vi "counter.vi"(7 "Fun":enum16{"Count", "Init"}(ring), 10 "INIT VALUE":dbl format="%#_13g") -> (2 "Numeric":dbl)   [LabVIEW 2015]
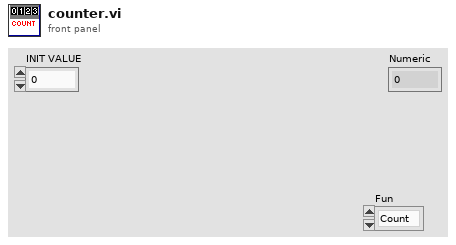
[diagram p1: front panel]
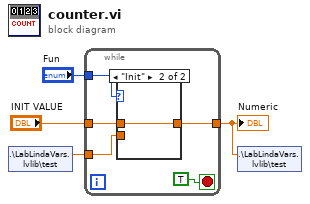
[diagram p0: block diagram]
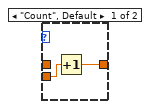
[diagram p2: hidden frame]
diagram:
  n1 = shared-variable ".\\LabLindaVars.lvlib\\test"() -> (w1:dbl)  [unwired: 1 in, 1 out]
  n2 = while {
    tunnel: "Fun" -> [w6]
    tunnel: "INIT VALUE" -> [w5]
    tunnel: w1 -> [w7]
    tunnel: [w8] -> w2
    stop <- TRUE stop-if-true
    n3 = case shown="\"Init\"" w6 {
      tunnel: [w11 w12] -> w8
      tunnel: w7 -> [w10 _]
      tunnel: w5 -> [_ w12]
      frame "Count", Default {
        n4 = Increment(x=w10) -> (x+1=w11:dbl)
      }
      frame "Init" {
      }
    }
  }
  "Numeric" <- w2
  n5 = shared-variable ".\\LabLindaVars.lvlib\\test"(w2) -> ()  [unwired: 1 in, 1 out]
